vi "Time_Interval.vi"() -> ()   [LabVIEW 2017, in "Examples.lvlib"]
uses:
  Examples.lvlib
panel:
  in  "Set Start Time (s)":dbl
  out "Voltage Waveform Chart  Logging":sgl(graph)
  in  "Stop Button":bool
  out "Logging?":bool
  out "Voltage Waveform Chart":sgl(graph)
  in  "Delay Time (s)":dbl=2.0
  in  "Start Time":timestamp
  in  "Stop Time":timestamp
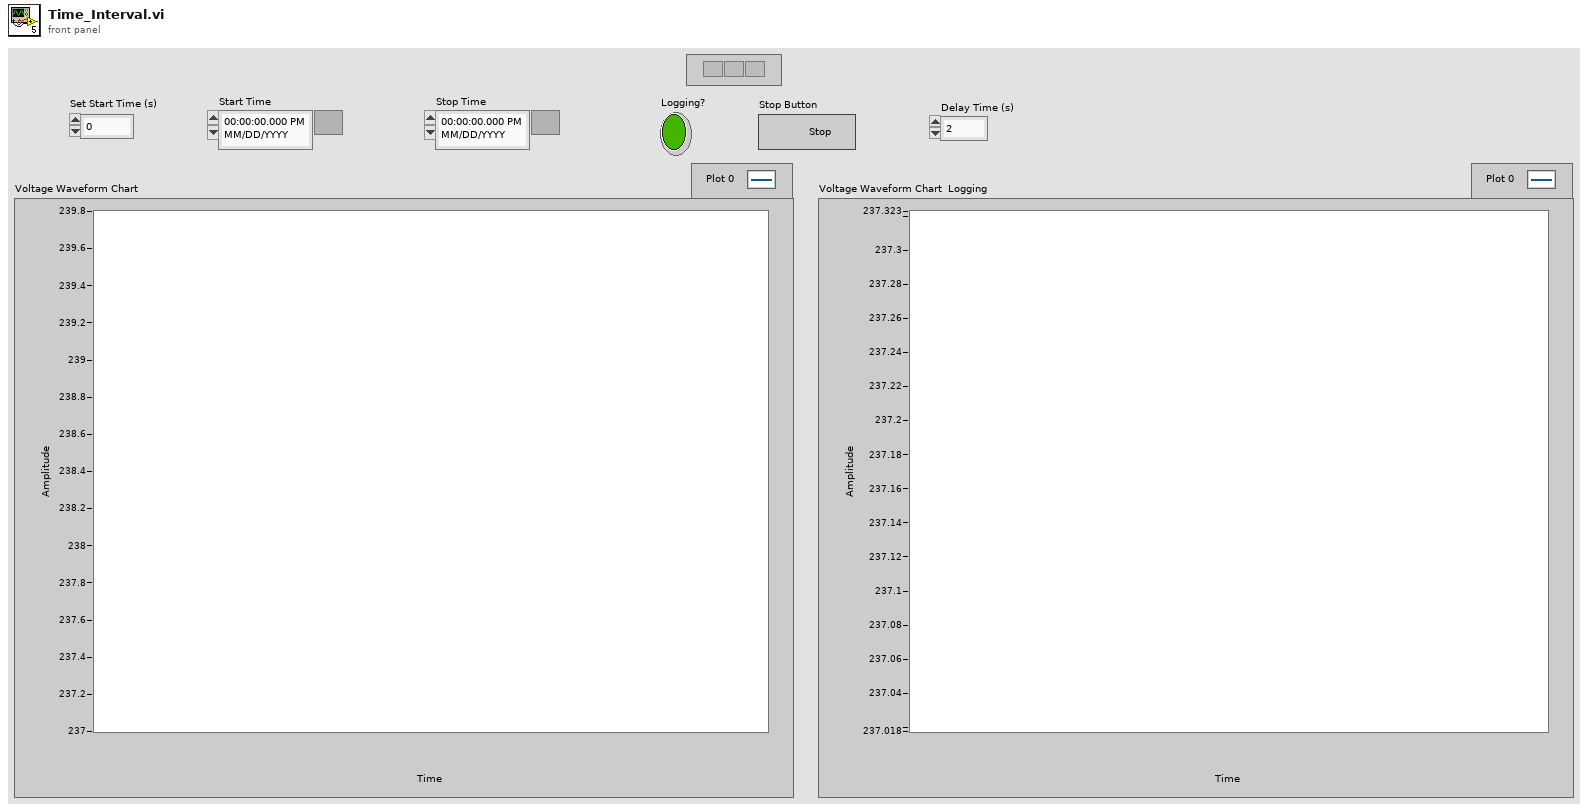
[diagram p1: front panel]
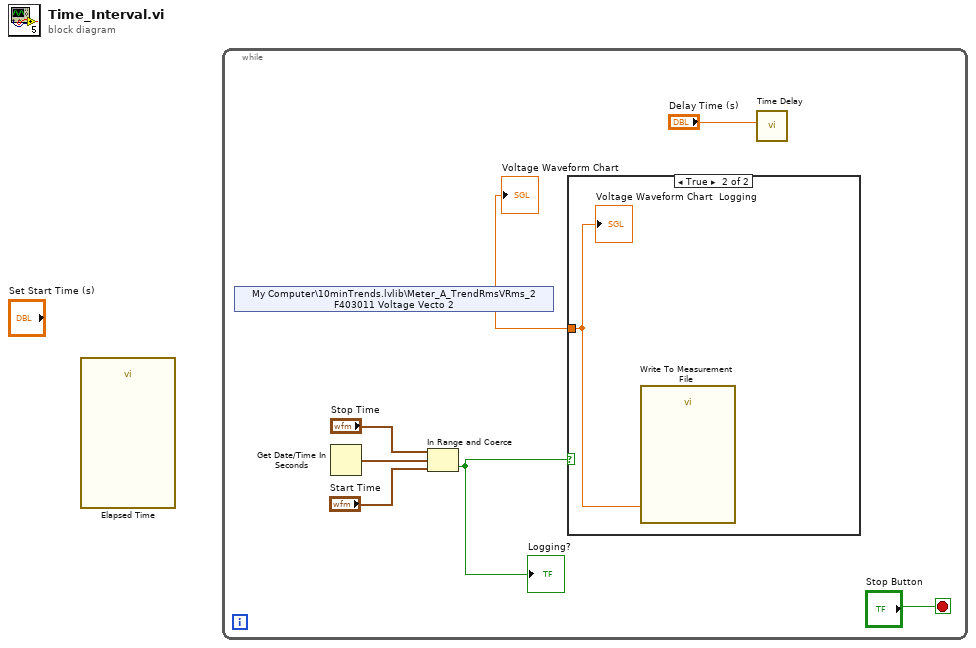
[diagram p0: block diagram]
diagram:
  n1 = call "Elapsed Time"() -> ()  [unwired: 12 in, 8 out]
  n2 = while {
    stop <- "Stop Button" stop-if-true
    n3 = shared-variable "My Computer\\10minTrends.lvlib\\Meter_A_TrendRmsVRms_2 F403011 Voltage Vecto 2"() -> (w1:sgl)  [unwired: 1 in, 1 out]
    "Voltage Waveform Chart" <- w1
    n4 = Get Date/Time In Seconds() -> (seconds since 1Jan1904=w5:timestamp)
    n5 = In Range and Coerce(upper limit="Stop Time", x=w5, lower limit="Start Time") -> (In Range?=w2:bool)  [unwired: 1 out]
    "Logging?" <- w2
    n6 = case shown="True" w2 {
      tunnel: w1 -> [_ w8]
      frame False {
      }
      frame True {
        n7 = call "Write To Measurement File"("Signals"=w8) -> ()  [unwired: 16 in, 3 out]
        "Voltage Waveform Chart  Logging" <- w8
      }
    }
    n8 = call "Time Delay"("Delay Time (s)"="Delay Time (s)") -> ()  [unwired: 10 in, 1 out]
  }
